vi "myRIO_BRig_RT__Case_Exp_State_endTrial2.vi"(6 "input_dataExp":u16[](array[numeric]), 9 "input_spout":enum16{"Left", "Right"}(ring), 10 "input_dataTrial":u16[][](array[numeric]), 11 "input_dataCurrent":u16[](array[numeric])) -> (2 "output_dataTrial":u16[][](array[numeric]), 3 "output_dataCurrent":u16[](array[numeric]))   [LabVIEW 2014]
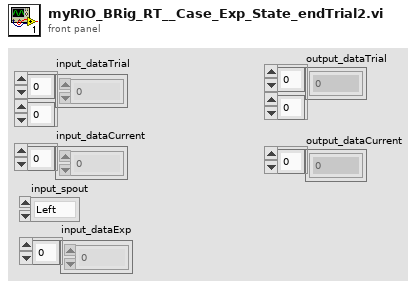
[diagram p1: front panel]
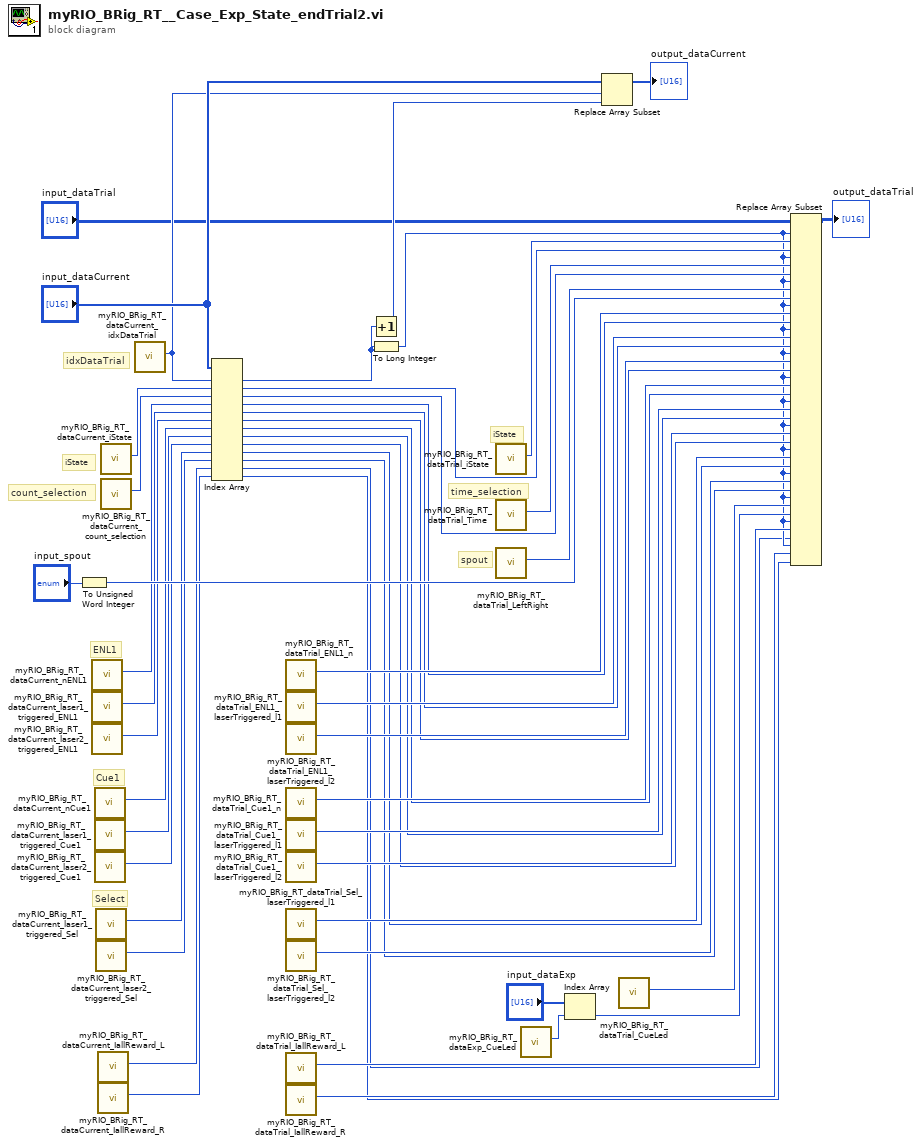
[diagram p0: block diagram]
diagram:
  # "Select"
  # "Cue1"
  # "ENL1"
  # "time_selection"
  # "spout"
  # "count_selection"
  # "iState"
  # "idxDataTrial"
  # "iState"
  n1 = To Unsigned Word Integer(number="input_spout") -> (unsigned 16bit integer=w36:u16)
  n2 = call "myRIO_BRig_RT_dataCurrent_nENL1.vi"() -> ("output_nENL1"=w35:i32)  [unwired: 11 in]
  n3 = call "myRIO_BRig_RT_dataCurrent_laser1_triggered_ENL1.vi"() -> ("output_laser1_triggered_ENL1"=w34:i32)  [unwired: 11 in]
  n4 = call "myRIO_BRig_RT_dataCurrent_laser2_triggered_ENL1.vi"() -> ("output_laser2_triggered_ENL1"=w12:i32)  [unwired: 11 in]
  n5 = call "myRIO_BRig_RT_dataCurrent_nCue1.vi"() -> ("output_nCue1"=w33:i32)  [unwired: 11 in]
  n6 = call "myRIO_BRig_RT_dataCurrent_laser1_triggered_Cue1.vi"() -> ("output_laser1_triggered_Cue1"=w32:i32)  [unwired: 11 in]
  n7 = call "myRIO_BRig_RT_dataCurrent_laser2_triggered_Cue1.vi"() -> ("output_laser2_triggered_Cue1"=w13:i32)  [unwired: 11 in]
  n8 = call "myRIO_BRig_RT_dataCurrent_laser1_triggered_Sel.vi"() -> ("output_laser1_triggered_Selection"=w31:i32)  [unwired: 11 in]
  n9 = call "myRIO_BRig_RT_dataCurrent_laser2_triggered_Sel.vi"() -> ("output_laser2_triggered_Selection"=w30:i32)  [unwired: 11 in]
  n10 = call "myRIO_BRig_RT_dataCurrent_IallReward_L.vi"() -> ("output_IallReward_L"=w7:i32)  [unwired: 11 in]
  n11 = call "myRIO_BRig_RT_dataCurrent_IallReward_R.vi"() -> ("output_IallReward_R"=w6:i32)  [unwired: 11 in]
  n12 = call "myRIO_BRig_RT_dataCurrent_iState.vi"() -> ("output_iState"=w51:i32)  [unwired: 11 in]
  n13 = call "myRIO_BRig_RT_dataCurrent_count_selection.vi"() -> ("output_count_generic"=w47:i32)  [unwired: 11 in]
  n14 = call "myRIO_BRig_RT_dataCurrent_idxDataTrial.vi"() -> ("output_idxDataTrial"=w45:i32)  [unwired: 11 in]
  n15 = Index Array(array="input_dataCurrent", index #1=w45, index #2=w51, index #3=w47, index #4=w35, index #5=w34, index #6=w12, index #7=w33, index #8=w32, index #9=w13, index #10=w31, index #11=w30, index #12=w7, index #13=w6) -> (element #1=w44:u16, element #2=w40:u16, element #3=w38:u16, element #4=w26:u16, element #5=w25:u16, element #6=w24:u16, element #7=w20:u16, element #8=w19:u16, element #9=w18:u16, element #10=w15:u16, element #11=w14:u16, element #12=w3:u16, element #13=w1:u16)
  n16 = call "myRIO_BRig_RT_dataTrial_ENL1_n.vi"() -> ("output_ENL1_n"=w29:i32)  [unwired: 11 in]
  n17 = call "myRIO_BRig_RT_dataTrial_ENL1_laserTriggered_l1.vi"() -> ("output_ENL1_laserTriggered_l1"=w28:i32)  [unwired: 11 in]
  n18 = call "myRIO_BRig_RT_dataTrial_ENL1_laserTriggered_l2.vi"() -> ("output_ENL1_laserTriggered_l2"=w27:i32)  [unwired: 11 in]
  n19 = call "myRIO_BRig_RT_dataTrial_Cue1_n.vi"() -> ("output_Cue1_n"=w23:i32)  [unwired: 11 in]
  n20 = call "myRIO_BRig_RT_dataTrial_Cue1_laserTriggered_l1.vi"() -> ("output_Cue1_laserTriggered_l1"=w22:i32)  [unwired: 11 in]
  n21 = call "myRIO_BRig_RT_dataTrial_Cue1_laserTriggered_l2.vi"() -> ("output_Cue1_laserTriggered_l2"=w21:i32)  [unwired: 11 in]
  n22 = call "myRIO_BRig_RT_dataTrial_Sel_laserTriggered_l1.vi"() -> ("output_Sel_laserTriggered_l1"=w17:i32)  [unwired: 11 in]
  n23 = call "myRIO_BRig_RT_dataTrial_Sel_laserTriggered_l2.vi"() -> ("output_Sel_laserTriggered_l2"=w16:i32)  [unwired: 11 in]
  n24 = call "myRIO_BRig_RT_dataTrial_IallReward_L.vi"() -> ("output_I_allReward_L"=w5:i32)  [unwired: 11 in]
  n25 = call "myRIO_BRig_RT_dataTrial_IallReward_R.vi"() -> ("output_I_allReward_R"=w2:i32)  [unwired: 11 in]
  n26 = Increment(x=w44) -> (x+1=w48:u16)
  n27 = To Long Integer(number=w44) -> (32bit integer=w4:i32)
  n28 = call "myRIO_BRig_RT_dataTrial_iState.vi"() -> ("output_iState"=w41:i32)  [unwired: 11 in]
  n29 = call "myRIO_BRig_RT_dataTrial_Time.vi"() -> ("output_Time"=w39:i32)  [unwired: 11 in]
  n30 = call "myRIO_BRig_RT_dataTrial_LeftRight.vi"() -> ("output_LeftRight"=w37:i32)  [unwired: 11 in]
  n31 = call "myRIO_BRig_RT_dataExp_CueLed.vi"() -> ("output_CueLed"=w10:i32)  [unwired: 11 in]
  n32 = Index Array(array="input_dataExp", index=w10) -> (element=w8:u16)
  n33 = Replace Array Subset(array="input_dataCurrent", new element=w48, index=w45) -> (→"output_dataCurrent":u16[])
  n34 = call "myRIO_BRig_RT_dataTrial_CueLed.vi"() -> ("output_CueLed"=w9:i32)  [unwired: 11 in]
  n35 = Replace Array Subset(array="input_dataTrial", new element #1=w40, index (row) #1=w4, index (col) #1=w41, new element #2=w38, index (row) #2=w4, index (col) #2=w39, new element #3=w36, index (row) #3=w4, index (col) #3=w37, new element #4=w26, index (row) #4=w4, index (col) #4=w29, new element #5=w25, index (row) #5=w4, index (col) #5=w28, new element #6=w24, index (row) #6=w4, index (col) #6=w27, new element #7=w20, index (row) #7=w4, index (col) #7=w23, new element #8=w19, index (row) #8=w4, index (col) #8=w22, new element #9=w18, index (row) #9=w4, index (col) #9=w21, new element #10=w15, index (row) #10=w4, index (col) #10=w17, new element #11=w14, index (row) #11=w4, index (col) #11=w16, new element #12=w8, index (row) #12=w4, index (col) #12=w9, new element #13=w3, index (row) #13=w4, index (col) #13=w5, new element #14=w1, index (row) #14=w4, index (col) #14=w2) -> (→"output_dataTrial":u16[][])
